vi "Main.vi"(11 "Module Admin":refnum<class "Delacor_lib_QMH_Module Admin.lvclass">) -> ()   [LabVIEW 2019, in "Settings Editor.lvlib"]
doc: "This template is based off of the Queued Message Handler design pattern and the Queued Message Handler project template that ships with LabVIEW.\n\nThe main difference is that the queue is private to this module and communication between modules is performed via Broadcast and Request events.\n\nRequest events are wrapped in public API methods and are handled in the Event Handling Loop (EHL) of this VI. Any module can register for Broadcast events sent by this module. The EHL generates messages based on user interface actions.\n\nThe Message Handling Loop (MHL) processes messages generated by the EHL, or by other messages. The messages are string values, so new messages can be added easily to the Message Cases case structure in the MHL. Each message cluster can also provide an optional value for Message Data, which is a variant that can be converted to whatever message-specific data is required.\n_____\nBased on Delacor QMH Project Template 4.0.0.47.\n_____\nBased on Delacor QMH Project Template 5.0.0.82."
uses:
  Settings Editor.lvlib
  <vilib>/Delacor/Delacor QMH/Libraries/Module Admin_class/Delacor_lib_QMH_Module Admin.lvclass
  Module Data--cluster.ctl
  Settings--cluster.ctl
  Stop Argument--cluster.ctl
  <vilib>/Delacor/Delacor QMH/Libraries/Message Queue_class/Delacor_lib_QMH_Message Queue.lvclass/Delacor_lib_QMH_Message Queue.ctl
  Update Application Settings Argument--cluster.ctl
  Update Application Settings (Reply Payload)--cluster.ctl
  <vilib>/Delacor/Delacor QMH/Libraries/Module Admin_class/Delacor_lib_QMH_Module Admin.lvclass/Delacor_lib_QMH_Module Admin.ctl
  <vilib>/Utility/miscctls.llb/LVPointTypeDef.ctl
  <vilib>/Delacor/Delacor QMH/Libraries/Message Queue_class/Delacor_lib_QMH_Enqueue Message (Single).vi
  <vilib>/Delacor/Delacor QMH/Libraries/Module Admin_class/Delacor_lib_QMH_Get External Launch.vi
  <vilib>/Utility/error.llb/Error Cluster From Error Code.vi
  <vilib>/ErrorRing/Error Ring.xnode
  <vilib>/Delacor/Delacor QMH/Libraries/Message Queue_class/Delacor_lib_QMH_Message Queue.lvclass
panel:
  in  "Min Value":dbl
  in  "Max Value":dbl
  in  "Analog Input Channel":refnum<k21>
  in  "Cancel":bool
  in  "OK":bool
  in  "Log File Base Path":path
  out "error out":errorcluster
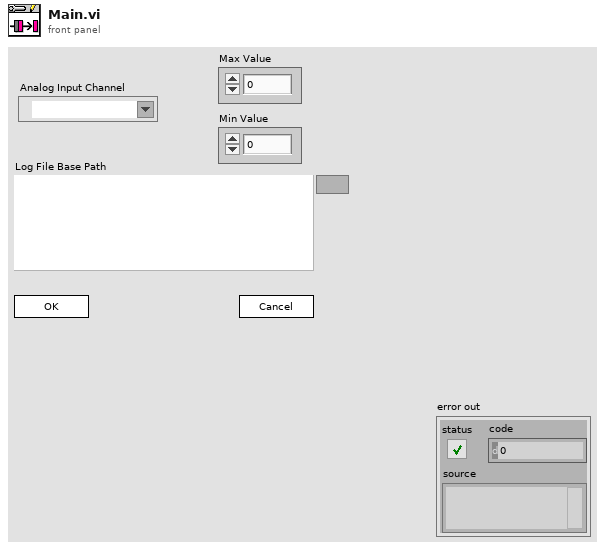
[diagram p1: front panel]
types:
  T1 = typedef "Settings Editor.lvlib/Request Events--cluster.ctl" = cluster{"Stop Module":refnum<user-event>, "Show Panel":refnum<user-event>, "Hide Panel":refnum<user-event>, "Get Module Execution Status":refnum<user-event>, "Show Diagram":refnum<user-event>, "Update Application Settings":refnum<user-event>}
  T2 = typedef "Settings Editor.lvlib/Module Data--cluster.ctl" = cluster{"Settings":T3}
  T3 = typedef "Settings Editor.lvlib/Settings--cluster.ctl" = cluster{"Log File Base Path":path, "Analog Input Channel":refnum<k21>, "Max Value":dbl, "Min Value":dbl}
  T4 = enum32{"invalid lock state", "Not Locked", "Locked (No Password)", "Password-protected"}
  T5 = typedef "Settings Editor.lvlib/Stop Argument--cluster.ctl" = cluster{"Origin":string, "Exit via Stop Module Req?":bool, "Wait for Module to stop?":bool}
  T6 = typedef "Settings Editor.lvlib/Update Application Settings Argument--cluster.ctl" = cluster{"Wait Notifier":refnum<notifier>, "wait for reply":bool}
  T7 = typedef "LVPointTypeDef.ctl" = cluster{"Horizontal":i16, "Vertical":i16}
  T8 = enum32{"Invalid", "Standard", "Closed", "Hidden", "Minimized", "Maximized"}
  T9 = typedef "Settings Editor.lvlib/Update Application Settings (Reply Payload)--cluster.ctl" = cluster{"Settings":T3, "Update Settings_error":errorcluster}
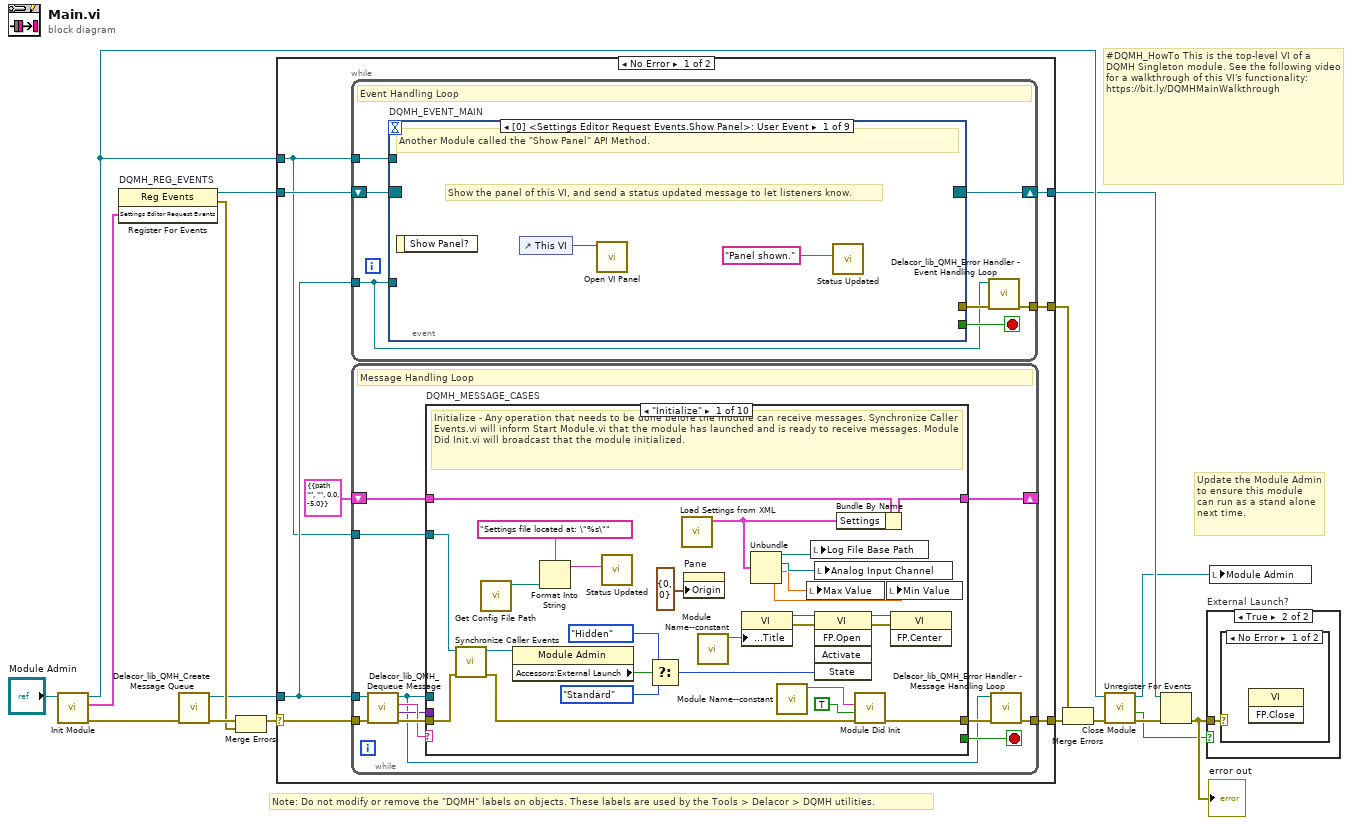
[diagram p0: block diagram]
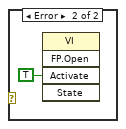
[diagram p3: hidden frame]
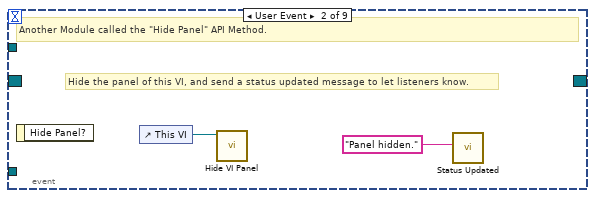
[diagram p4: hidden frame]
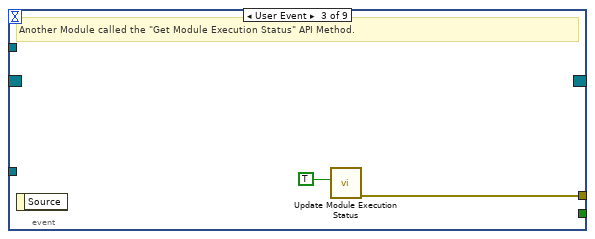
[diagram p5: hidden frame]
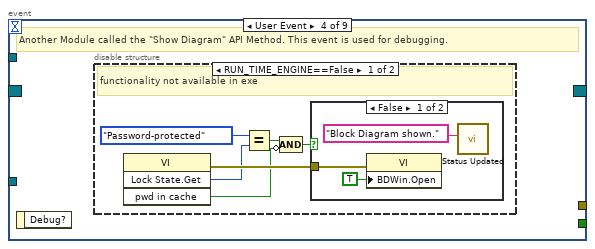
[diagram p6: hidden frame]
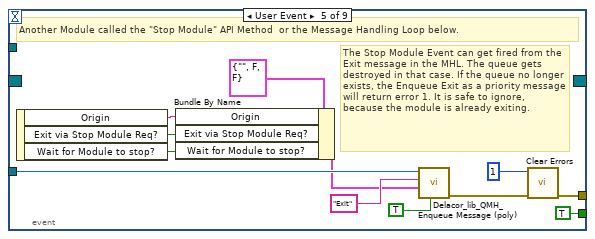
[diagram p9: hidden frame]
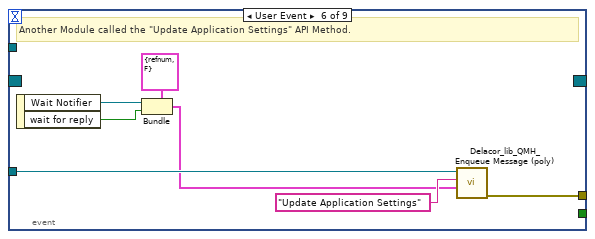
[diagram p10: hidden frame]
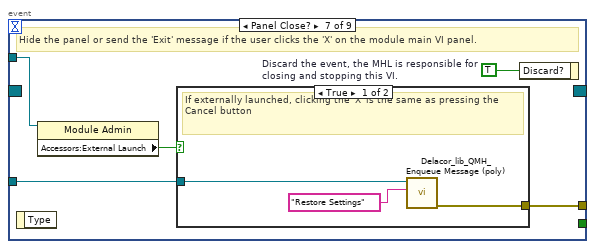
[diagram p11: hidden frame]
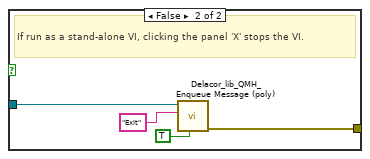
[diagram p12: hidden frame]
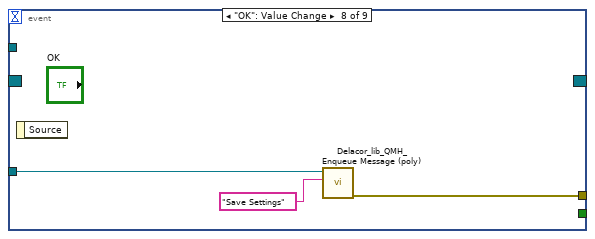
[diagram p13: hidden frame]
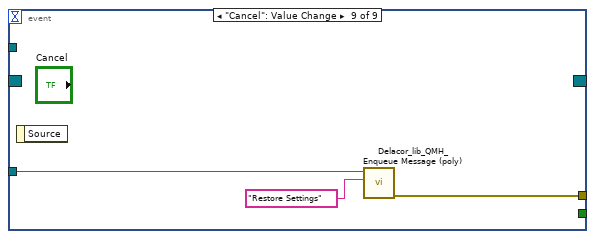
[diagram p14: hidden frame]
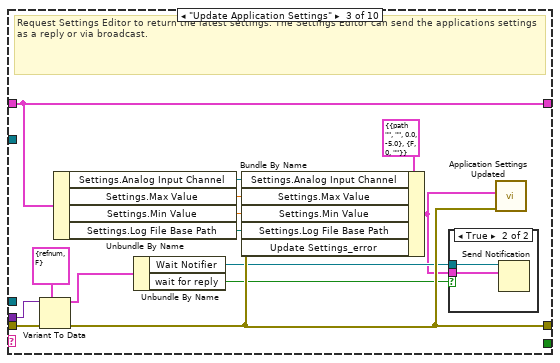
[diagram p16: hidden frame]
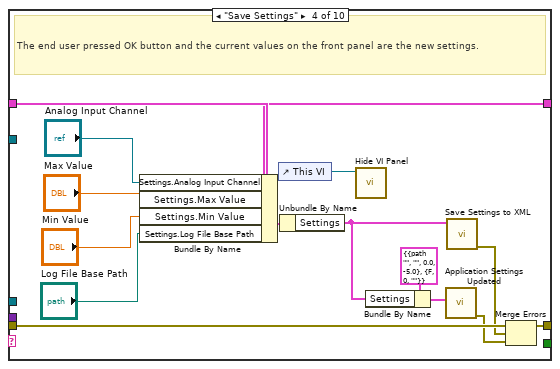
[diagram p18: hidden frame]
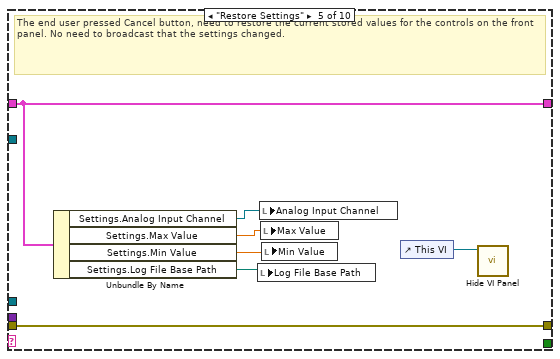
[diagram p19: hidden frame]
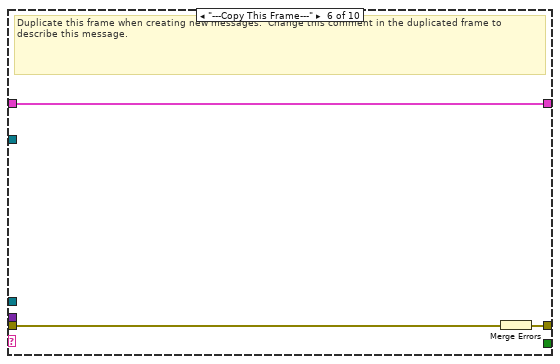
[diagram p20: hidden frame]
diagram:
  # "#DQMH_HowTo This is the top-level VI of a DQMH Singleton module. See the following video for a walkthrough of this VI's functionality: https://bit.ly/DQMHMainWalkthrough"
  # "Note: Do not modify or remove the \"DQMH\" labels on objects. These labels are used by the Tools > Delacor > DQMH utilities."
  # "Update the Module Admin to ensure this module can run as a stand alone next time."
  n1 = call "Init Module.vi"("Singleton Module Admin in"="Module Admin") -> ("error out"=w16:errorcluster, "Settings Editor Request Events"=w5:T1, "Singleton Module Admin out"=w8:refnum<class "Delacor_lib_QMH_Module Admin.lvclass">)  [unwired: 8 in]
  n2 = register-events "DQMH_REG_EVENTS"(w5) -> (reference out=w6:refnum<event-registration>, error out=w9:errorcluster)  [unwired: 2 in]
  n3 = call <vilib>:"Delacor_lib_QMH_Create Message Queue.vi"("error in"=w16) -> ("error out"=w11:errorcluster, "Message Queue"=w4:refnum<class "Delacor_lib_QMH_Message Queue.lvclass">)  [unwired: 9 in]
  n4 = Merge Errors(w11, w9) -> (w10:errorcluster)
  n5 = case shown="No Error" w10 {
    selector: w10 -> [w23 w215]
    tunnel: [w25 w214] -> w17
    tunnel: [w22 w221] -> w7
    tunnel: w6 -> [w20 w221]
    tunnel: w4 -> [w19 w216]
    tunnel: [w24 _] -> w14
    tunnel: w8 -> [w18 w217]
    frame No Error {
      n6 = while {
        tunnel: w19 -> [w26]
        shift-right: [w29] -> w22
        shift-left: w20 -> [w30]
        tunnel: [w31] -> w24
        tunnel: w18 -> [w27]
        stop <- w28 stop-if-true
        # "Event Handling Loop"
        n7 = event "DQMH_EVENT_MAIN" shown="[0] <Settings Editor Request Events.Show Panel>: User Event" {
          selector: w30 -> [_ _ _ _ _ _ _ _ _]
          dyn-events: [_ _ _ _ _ _ _ _ _] -> w29
          timeout: _ -> [_ _ _ _ _ _ _ _ _]
          tunnel: [_ _ _ _ TRUE ("Discard?") _ _ _ _] -> w28
          tunnel: w26 -> [_ _ _ _ w55 w66 w69 w79 w83]
          tunnel: [_ _ w38 _ w58 w62 w71 w80 w82] -> w32
          tunnel: w27 -> [_ _ _ _ _ _ w68 _ _]
          event User Event {
            # "Show the panel of this VI, and send a status updated message to let listeners know."
            # "Another Module called the \"Show Panel\" API Method."
            n8 = event-data() -> ()  [unwired: 1 in, 1 out]
            n9 = control-ref of="This VI"() -> (w34:refnum<vi>)
            n10 = call "Open VI Panel.vi"("VI"=w34) -> ()  [unwired: 10 in, 1 out]
            n11 = call "Status Updated.vi"("Status"="Panel shown." ("format string")) -> ()  [unwired: 10 in, 1 out]
          }
          event User Event {
            # "Hide the panel of this VI, and send a status updated message to let listeners know."
            # "Another Module called the \"Hide Panel\" API Method."
            n12 = event-data() -> ()  [unwired: 1 in, 1 out]
            n13 = control-ref of="This VI"() -> (w36:refnum<vi>)
            n14 = call "Hide VI Panel.vi"("VI"=w36) -> ()  [unwired: 10 in, 1 out]
            n15 = call "Status Updated.vi"("Status"="Panel hidden." ("format string")) -> ()  [unwired: 10 in, 1 out]
          }
          event User Event {
            # "Another Module called the \"Get Module Execution Status\" API Method."
            n16 = event-data() -> ()  [unwired: 1 in, 1 out]
            n17 = call "Update Module Execution Status.vi"("Running?"=TRUE) -> ("error out"=w38:errorcluster)  [unwired: 10 in]
          }
          event User Event {
            # "Another Module called the \"Show Diagram\" API Method. This event is used for debugging."
            n18 = event-data() -> ()  [unwired: 1 in, 1 out]
            n19 = disable-structure shown="RUN_TIME_ENGINE==False" {
              frame condition #0 (active) {
                # "functionality not available in exe"
                n20 = invoke class="VI" method="Lock State.Get"() -> (error out=w44:errorcluster, "Get Lock State"=w43:T4, "pwd in cache"=w40:bool)  [unwired: 4 in, 1 out]
                n21 = Equal?(x=T4."Password-protected", y=w43) -> (x = y?=w41:bool)
                n22 = Compound Arithmetic op=AND(w41, invert w40) -> (w39:bool)
                n23 = case shown="False" w39 {
                  tunnel: w44 -> [w47 _]
                  frame False {
                    n24 = property class="VI"(error in=w47, "BDWin.Open"=TRUE ("Block Diagram Window:Open")) -> ()  [unwired: 1 in, 2 out]
                    n25 = call "Status Updated.vi"("Status"="Block Diagram shown." ("format string")) -> ()  [unwired: 10 in, 1 out]
                  }
                  frame True {
                    # "Password-protected VI, and the password is not in the cache. Do not show the diagram."
                  }
                }
              }
              frame condition #1 {
              }
            }
          }
          event User Event {
            # "The Stop Module Event can get fired from the Exit message in the MHL. The queue gets destroyed in that case. If the queue no longer exists, the Enqueue Exit as a priority message will return error 1. It is safe to ignore, because the module is already exiting."
            # "Another Module called the \"Stop Module\" API Method  or the Message Handling Loop below."
            n26 = event-data() -> ("Origin"=w48:string, "Exit via Stop Module Req?"=w51:bool, "Wait for Module to stop?"=w50:bool)  [unwired: 1 in]
            n27 = Bundle By Name(cluster=T5 {"Origin"="", "Exit via Stop Module Req?"=FALSE, "Wait for Module to stop?"=FALSE} ("Stop Argument"), "Origin"=w48, "Exit via Stop Module Req?"=w51, "Wait for Module to stop?"=w50) -> (w49:T5)
            n28 = call-poly <vilib>:"Delacor_lib_QMH_Enqueue Message (poly).vi"("Priority Message? (F)"=TRUE, "Message Data"=w49, "Message"="Exit", "Message Queue in"=w55) -> ("error out"=w59:errorcluster)  [unwired: 6 in, 1 out]
            n29 = call <vilib>:"Clear Errors.vi"("error in (no error)"=w59, "specific error code to clear (0: all)"=1) -> ("error out"=w58:errorcluster)  [unwired: 4 in, 1 out]
          }
          event User Event {
            # "Another Module called the \"Update Application Settings\" API Method."
            n30 = event-data() -> ("Wait Notifier"=w61:refnum<notifier>, "wait for reply"=w60:bool)  [unwired: 1 in]
            n31 = Bundle(cluster=T6 {"Wait Notifier"=refnum, "wait for reply"=FALSE} ("Update Application Settings Argument"), "Wait Notifier"=w61, "wait for reply"=w60) -> (w63:T6)
            n32 = call-poly <vilib>:"Delacor_lib_QMH_Enqueue Message (poly).vi"("Message Data"=w63, "Message"="Update Application Settings", "Message Queue in"=w66) -> ("error out"=w62:errorcluster)  [unwired: 7 in, 1 out]
          }
          event Panel Close? {
            w70 = TRUE  # Discard the event, the MHL is responsible for closing and stopping this VI.
            # "Hide the panel or send the 'Exit' message if the user clicks the 'X' on the module main VI panel."
            n33 = event-data() -> ()  [unwired: 1 in, 1 out]
            n34 = property class="Module Admin"(reference=w68) -> ("Accessors:External Launch"=w67:bool)  [unwired: 1 in, 2 out]
            n35 = case shown="True" w67 {
              tunnel: w69 -> [w73 w77]
              tunnel: [w72 w78] -> w71
              frame True {
                # "If externally launched, clicking the 'X' is the same as pressing the Cancel button"
                n36 = call-poly <vilib>:"Delacor_lib_QMH_Enqueue Message (poly).vi"("Message"="Restore Settings", "Message Queue in"=w73) -> ("error out"=w72:errorcluster)  [unwired: 8 in, 1 out]
              }
              frame False {
                # "If run as a stand-alone VI, clicking the panel 'X' stops the VI."
                n37 = call-poly <vilib>:"Delacor_lib_QMH_Enqueue Message (poly).vi"("Priority Message? (F)"=TRUE, "Message"="Exit", "Message Queue in"=w77) -> ("error out"=w78:errorcluster)  [unwired: 7 in, 1 out]
              }
            }
            n38 = event-data("Discard?"=w70) -> ()  [unwired: 1 in, 1 out]
          }
          event "OK": Value Change {
            n39 = event-data() -> ()  [unwired: 1 in, 1 out]
            n40 = call-poly <vilib>:"Delacor_lib_QMH_Enqueue Message (poly).vi"("Message"="Save Settings", "Message Queue in"=w79) -> ("error out"=w80:errorcluster)  [unwired: 8 in, 1 out]
          }
          event "Cancel": Value Change {
            n41 = event-data() -> ()  [unwired: 1 in, 1 out]
            n42 = call-poly <vilib>:"Delacor_lib_QMH_Enqueue Message (poly).vi"("Message"="Restore Settings", "Message Queue in"=w83) -> ("error out"=w82:errorcluster)  [unwired: 8 in, 1 out]
          }
        }
        n43 = call-dynamic "Delacor_lib_QMH_Error Handler - Event Handling Loop.vi"("error in"=w32, "Message Queue in"=w26) -> ("dup error in"=w31:errorcluster)  [unwired: 8 in, 1 out]
      }
      n44 = while {
        tunnel: w19 -> [w87]
        shift-right: [w91] -> _
        shift-left: T2 {"Settings"={"Log File Base Path"=path "", "Analog Input Channel"="", "Max Value"=0.0, "Min Value"=-5.0}} ("Data Cluster") -> [w92]
        tunnel: w23 -> [w95]
        tunnel: [w93] -> w25
        tunnel: w18 -> [w85]
        stop <- w90 stop-if-true
        # "Message Handling Loop"
        n45 = call-dynamic "Delacor_lib_QMH_Dequeue Message.vi"("error in"=w95, "Message Queue in"=w87) -> ("error out"=w94:errorcluster, "Message Data"=w88:variant, "Message"=w89:string, "Message Queue out"=w86:refnum<class "Delacor_lib_QMH_Message Queue.lvclass">)  [unwired: 6 in]
        n46 = case "DQMH_MESSAGE_CASES" shown="\"Initialize\"" w89 {
          selector: w89 -> [_ _ _ _ _ _ _ _ _ w201]
          tunnel: w86 -> [_ _ _ _ _ _ _ w171 w193 _]
          tunnel: w94 -> [w122 w125 w138 w147 w162 w165 w167 w178 w199 w203]
          tunnel: [w120 w125 w139 w148 w162 w164 w167 w174 w196 w204] -> w96
          tunnel: w92 -> [w111 w124 w132 w155 w161 w163 w166 w173 w192 w202]
          tunnel: [w110 w124 w132 w153 w161 w163 w166 w173 w192 w202] -> w91
          tunnel: [_ _ _ _ _ _ _ _ w191 _] -> w90
          tunnel: w88 -> [_ _ w137 _ _ _ _ w172 w190 _]
          tunnel: w85 -> [w112 _ _ _ _ _ _ w170 w185 _]
          frame "Initialize" {
            # "Initialize - Any operation that needs to be done before the module can receive messages. Synchronize Caller Events.vi will inform Start Module.vi that the module has launched and is ready to receive messages. Module Did Init.vi will broadcast that the module initialized."
            n47 = call "Synchronize Caller Events.vi"("error in (no error)"=w122, "Singleton Module Admin in"=w112) -> ("error out"=w121:errorcluster, "Singleton Module Admin out"=w107:refnum<class "Delacor_lib_QMH_Module Admin.lvclass">)  [unwired: 8 in]
            n48 = call "Get Config File Path.vi"() -> ("XML File Path"=w104:path)  [unwired: 10 in, 1 out]
            n49 = property class="Module Admin"(reference=w107) -> ("Accessors:External Launch"=w116:bool)  [unwired: 1 in, 2 out]
            n50 = Format Into String(format string="Settings file located at: \"%s\"", w104) -> (resulting string=w103:string)  [unwired: 2 in, 1 out]
            n51 = call "Status Updated.vi"("Status"=w103) -> ()  [unwired: 10 in, 1 out]
            n52 = Select(t=T8."Hidden" ("State"), s=w116, f=T8."Standard" ("State")) -> (s? t:f=w113:T8)
            n53 = call "Load Settings from XML.vi"() -> ("Settings Out"=w101:T3)  [unwired: 10 in, 1 out]
            n54 = property on="Pane" class="Pane"("Origin"=T7 {"Horizontal"=0, "Vertical"=0}) -> ()  [unwired: 2 in, 2 out]
            n55 = call "Module Name--constant.vi"() -> ("Module Name"=w119:string)  [unwired: 11 in]
            n56 = property class="VI"("Front Panel.Title"=w119) -> (reference out=w118:refnum<vi>, error out=w105:errorcluster)  [unwired: 2 in]
            n57 = Unbundle(w101) -> ("Log File Base Path"=w100:path, "Analog Input Channel"=w99:refnum<k21>, "Max Value"=w98:dbl, "Min Value"=w97:dbl)
            n58 = call "Module Name--constant.vi"() -> ("Module Name"=w108:string)  [unwired: 11 in]
            n59 = local write "Max Value"(w98) -> ()
            n60 = local write "Log File Base Path"(w100) -> ()
            n61 = local write "Analog Input Channel"(w99) -> ()
            n62 = invoke class="VI" method="FP.Open"(reference=w118, error in=w105, "State"=w113) -> (reference out=w117:refnum<vi>, error out=w123:errorcluster)  [unwired: 2 in, 3 out]
            n63 = Bundle By Name(cluster=w111, "Settings"=w101) -> (w110:T2)
            n64 = call "Module Did Init.vi"("error in (no error)"=w121, "Initialized?"=TRUE, "Origin"=w108) -> ("error out"=w120:errorcluster)  [unwired: 8 in]
            n65 = local write "Min Value"(w97) -> ()
            n66 = invoke class="VI" method="FP.Center"(reference=w117, error in=w123) -> ()  [unwired: 1 in, 3 out]
          }
          frame "--- Module Specific ---" {
            # "Separator -- The following cases handle messages specific to this Module."
          }
          frame "Update Application Settings" {
            # "Request Settings Editor to return the latest settings. The Settings Editor can send the applications settings as a reply or via broadcast."
            n67 = Variant To Data(error in=w138, type=T6 {"Wait Notifier"=refnum, "wait for reply"=FALSE} ("Update Application Settings Argument"), Variant=w137) -> (data=w135:T6, error out=w139:errorcluster)
            n68 = Unbundle By Name(w132) -> ("Settings.Analog Input Channel"=w126:refnum<k21>, "Settings.Max Value"=w127:dbl, "Settings.Min Value"=w128:dbl, "Settings.Log File Base Path"=w130:path)
            n69 = Unbundle By Name(w135) -> ("Wait Notifier"=w134:refnum<notifier>, "wait for reply"=w133:bool)
            n70 = Bundle By Name(cluster=T9 {"Settings"={"Log File Base Path"=path "", "Analog Input Channel"="", "Max Value"=0.0, "Min Value"=-5.0}, "Update Settings_error"={"status"=FALSE, "code"=0, "source"=""}} ("Update Application Settings (Reply Payload)"), "Settings.Analog Input Channel"=w126, "Settings.Max Value"=w127, "Settings.Min Value"=w128, "Settings.Log File Base Path"=w130, "Update Settings_error"=w139) -> (w129:T9)
            n71 = case shown="True" w133 {
              tunnel: w134 -> [_ w141]
              tunnel: w129 -> [_ w140]
              frame False {
              }
              frame True {
                n72 = Send Notification(notification=w140, notifier=w141) -> ()  [unwired: 1 in, 2 out]
              }
            }
            n73 = call "Application Settings Updated.vi"("error in (no error)"=w139, "Reply Payload"=w129) -> ()  [unwired: 9 in, 1 out]
          }
          frame "Save Settings" {
            # "The end user pressed OK button and the current values on the front panel are the new settings."
            n74 = Bundle By Name(cluster=w155, "Settings.Analog Input Channel"="Analog Input Channel", "Settings.Max Value"="Max Value", "Settings.Min Value"="Min Value", "Settings.Log File Base Path"="Log File Base Path") -> (w153:T2)
            n75 = control-ref of="This VI"() -> (w154:refnum<vi>)
            n76 = Unbundle By Name(w153) -> ("Settings"=w149:T3)
            n77 = call "Hide VI Panel.vi"("VI"=w154) -> ()  [unwired: 10 in, 1 out]
            n78 = Bundle By Name(cluster=T9 {"Settings"={"Log File Base Path"=path "", "Analog Input Channel"="", "Max Value"=0.0, "Min Value"=-5.0}, "Update Settings_error"={"status"=FALSE, "code"=0, "source"=""}} ("Reply Payload"), "Settings"=w149) -> (w150:T9)
            n79 = call "Application Settings Updated.vi"("Reply Payload"=w150) -> ("error out"=w145:errorcluster)  [unwired: 10 in]
            n80 = call "Save Settings to XML.vi"("Settings"=w149) -> ("error out"=w146:errorcluster)  [unwired: 10 in]
            n81 = Merge Errors(w147, w146, w145) -> (w148:errorcluster)
          }
          frame "Restore Settings" {
            # "The end user pressed Cancel button, need to restore the current stored values for the controls on the front panel. No need to broadcast that the settings changed."
            n82 = Unbundle By Name(w161) -> ("Settings.Analog Input Channel"=w158:refnum<k21>, "Settings.Max Value"=w157:dbl, "Settings.Min Value"=w156:dbl, "Settings.Log File Base Path"=w160:path)
            n83 = local write "Log File Base Path"(w160) -> ()
            n84 = local write "Analog Input Channel"(w158) -> ()
            n85 = local write "Max Value"(w157) -> ()
            n86 = local write "Min Value"(w156) -> ()
            n87 = control-ref of="This VI"() -> (w159:refnum<vi>)
            n88 = call "Hide VI Panel.vi"("VI"=w159) -> ()  [unwired: 10 in, 1 out]
          }
          frame "---Copy This Frame---" {
            # "Duplicate this frame when creating new messages.  Change this comment in the duplicated frame to describe this message."
            n89 = Merge Errors(w165) -> (w164:errorcluster)
          }
          frame "--- Exit and Error Handling---" {
            # "Separator - The following cases handle errors and exit messages."
          }
          frame "Error" {
            # "Error - Check the error message data and respond accordingly. This message is sent by the \"Error Handler\" VIs at the end of each loop in this application."
            n90 = property class="Module Admin"(reference=w170) -> ("Accessors:External Launch"=w169:bool)  [unwired: 1 in, 2 out]
            n91 = Variant To Data(error in=w178, type=errorcluster {"status"=FALSE, "code"=0, "source"=""} ("error constant"), Variant=w172) -> (data=w179:errorcluster, error out=w176:errorcluster)
            n92 = call "Module Name--constant.vi"() -> ("Module Name"=w168:string)  [unwired: 11 in]
            n93 = call "Error Reported.vi"("Additional Information"=w168, "Error"=w179) -> ()  [unwired: 9 in, 1 out]
            n94 = case shown="False" w169 {
              tunnel: [w184 _] -> w175
              tunnel: w171 -> [w182 _]
              tunnel: w179 -> [w183 _]
              frame False {
                # "If the module is running standalone, then pop up an error dialog and call the \"Exit\" message."
                n95 = call <vilib>:"Simple Error Handler.vi"("error in (no error)"=w183) -> ()  [unwired: 4 in, 5 out]
                n96 = call-poly <vilib>:"Delacor_lib_QMH_Enqueue Message (poly).vi"("Priority Message? (F)"=TRUE, "Message"="Exit", "Message Queue in"=w182) -> ("error out"=w184:errorcluster)  [unwired: 7 in, 1 out]
              }
              frame True {
                # "If the module was launched externally, calling the Error Reported broadcast VI is the only action performed by the \"Error\" message. The module's caller can then process the error appropriately."
              }
            }
            n97 = Merge Errors(w176, w175) -> (w174:errorcluster)
            n98 = local write "error out"(w174) -> ()
          }
          frame "Exit" {
            w189 = 91  # 91: not all Exit messages will have an argument
            w191 = TRUE  # Stop the VI
            # "Release the message queue reference"
            # "Exit - Exit the application."
            n99 = Variant To Data(error in=w199, type=T5 {"Origin"="", "Exit via Stop Module Req?"=FALSE, "Wait for Module to stop?"=FALSE} ("Stop Argument"), Variant=w190) -> (data=w187:T5, error out=w195:errorcluster)
            n100 = call <vilib>:"Clear Errors.vi"("error in (no error)"=w195, "specific error code to clear (0: all)"=w189) -> ("error out"=w198:errorcluster)  [unwired: 4 in, 1 out]
            n101 = control-ref of="This VI"() -> (w186:refnum<vi>)
            n102 = call-dynamic "Delacor_lib_QMH_Release Message Queue.vi"("error in"=w198, "Message Queue"=w193) -> ("error out"=w197:errorcluster)  [unwired: 9 in]
            n103 = call "Handle Exit.vi"("Stop Argument"=w187, "Admin in"=w185, "VI reference"=w186) -> ("error out"=w194:errorcluster)  [unwired: 7 in, 1 out]
            n104 = Merge Errors(w197, w194) -> (w196:errorcluster)
          }
          frame Default {
            # "'Default' case only runs if there is a message that isn't defined in any of the other cases.  Output a programming error."
            n105 = call "Module Name--constant.vi"() -> ("Module Name"=w200:string)  [unwired: 11 in]
            n106 = xnode "Error Ring"("parameter 0"=w201, "parameter 1"=w200) -> ("error out"=w205:errorcluster)
            n107 = Merge Errors(w203, w205) -> (w204:errorcluster)
          }
        }
        n108 = call-dynamic "Delacor_lib_QMH_Error Handler - Message Handling Loop.vi"("error in"=w96, "Message Queue in"=w86) -> ("dup error in"=w93:errorcluster)  [unwired: 8 in, 1 out]
      }
    }
    frame Error {
      # "Synchronize Caller Events.vi will inform Start Module.vi that the module has launched and will let the code calling Start Module.vi register for broadcasts and would permit the caller receive the broadcast that an error occurred at launch time."
      n109 = call "Synchronize Caller Events.vi"("Singleton Module Admin in"=w217) -> ("error out"=w222:errorcluster)  [unwired: 9 in, 1 out]
      n110 = call-dynamic "Delacor_lib_QMH_Release Message Queue.vi"("error in"=w215, "Message Queue"=w216) -> ("error out"=w214:errorcluster)  [unwired: 9 in]
      n111 = call "Module Name--constant.vi"() -> ("Module Name"=w220:string)  [unwired: 11 in]
      n112 = Format Into String(format string="An error occurred during initialization. %s is no longer running.", w220) -> (resulting string=w218:string)  [unwired: 2 in, 1 out]
      n113 = Merge Errors(w214, w222) -> (w223:errorcluster)
      n114 = call "Error Reported.vi"("Additional Information"=w218, "Error"=w223) -> ()  [unwired: 9 in, 1 out]
    }
  }
  n115 = Merge Errors(w14, w17) -> (w13:errorcluster)
  n116 = call "Close Module.vi"("error in (no error)"=w13, "Module Admin in"=w8) -> ("error out"=w15:errorcluster, "External Launch"=w1:bool, "Module Admin out"=w2:refnum<class "Delacor_lib_QMH_Module Admin.lvclass">)  [unwired: 7 in]
  n117 = Unregister For Events(event registration refnum=w7, error in=w15) -> (error out=w12:errorcluster)
  "error out" <- w12
  n118 = case "External Launch?" shown="True" w1 {
    tunnel: w12 -> [_ w224]
    frame False {
    }
    frame True {
      n119 = case shown="No Error" w224 {
        frame No Error {
          n120 = invoke class="VI" method="FP.Close"() -> ()  [unwired: 3 in, 3 out]
        }
        frame Error {
          n121 = invoke class="VI" method="FP.Open"("Activate"=TRUE ("Activate?")) -> ()  [unwired: 4 in, 5 out]
        }
      }
    }
  }
  n122 = local write "Module Admin"(w2) -> ()
